vi "WriteKeys.vi"(8 "error in (no error)":errorcluster, 9 "Value":i32[](array[numeric]), 10 "Keys":string[](array[string]), 11 "Device in":refnum<class "Device.lvclass">) -> (0 "error out":errorcluster, 3 "Device out":refnum<class "Device.lvclass">)   [LabVIEW 2020, in "Device.lvlib" / "Device.lvclass"]
uses:
  Device.lvclass
  Device.lvclass/Device.ctl
  <vilib>/Utility/config.llb/Write Key (I32).vi
  <vilib>/Utility/config.llb/NI_LVConfig.lvlib
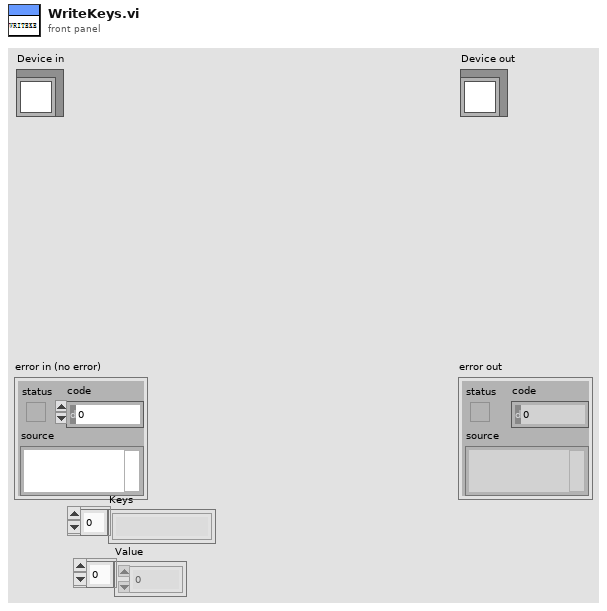
[diagram p1: front panel]
types:
  T1 = typedef "NI_LVConfig.lvlib/Config Data RefNum.ctl" = refnum<k1>
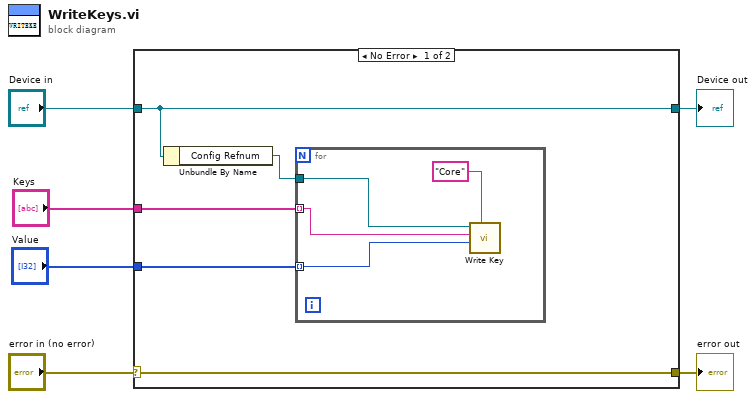
[diagram p0: block diagram]
diagram:
  n1 = case shown="No Error" "error in (no error)" {
    selector: "error in (no error)" -> [w11 w17]
    tunnel: [w11 w17] -> w5
    tunnel: [w10 w16] -> w3
    tunnel: "Device in" -> [w10 w16]
    tunnel: "Keys" -> [w8 _]
    tunnel: "Value" -> [w7 _]
    frame No Error {
      n2 = Unbundle By Name(w10) -> ("Config Refnum"=w9:T1)
      n3 = for {
        tunnel: w9 -> [w14]
        tunnel: w8 -> [w13] mode=indexing
        tunnel: w7 -> [w12] mode=indexing
        n4 = call-poly <vilib>:"Write Key.vi"("section"="Core", "value"=w12, "key"=w13, "refnum"=w14) -> ()  [unwired: 5 in, 3 out]
      }
    }
    frame Error {
    }
  }
  "error out" <- w5
  "Device out" <- w3
